vi "WS1050_AD7747_Init 36DUT.vi"(8 "error in":errorcluster) -> (0 "error out":errorcluster)   [LabVIEW 2012]
uses:
  WS_VCAP Driver 029/Source/WSVCAP Shell/Type Defs/WSVCAP SHL I2C DUT Mask Mode Enum.ctl
panel:
  # "Initialize AD7747 for Capacitance Measurement Mode"
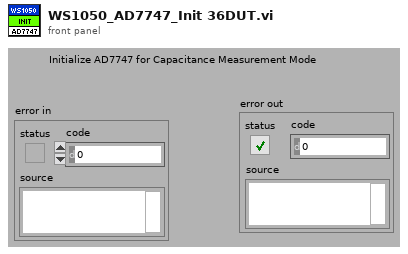
[diagram p1: front panel]
types:
  T1 = typedef "WSVCAP SHL I2C DUT Mask Mode Enum.ctl" = enum16{"Custom", "C1", "C2", "C3", "All"}
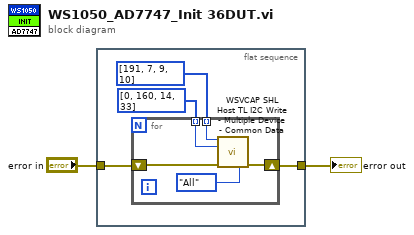
[diagram p0: block diagram]
diagram:
  n1 = flat-sequence {
    tunnel: "error in" -> [w6]
    tunnel: [w5] -> w2
    frame #0 {
      n2 = for {
        tunnel: u8[] [191, 7, 9, 10] -> [w9] mode=indexing
        tunnel: u8[] [0, 160, 14, 33] -> [w8] mode=indexing
        shift-right: [w11] -> w5
        shift-left: w6 -> [w10]
        n3 = call "WSVCAP SHL Host TL I2C Write - Multiple Device - Common Data.vi"("Sub Address"=w9, "Data Out [U8]"=w8, "error in"=w10, "DUT Mask Mode (All)"=WSVCAP_SHL_I2C_DUT_Mask_Mode_Enum."All") -> ("error out"=w11:errorcluster)  [unwired: 11 in]
      }
    }
  }
  "error out" <- w2
